vi "Login.vi"(5 "key":string="pGHs5Pd97hphPAMAKeEquwhT8aC4MC2e", 7 "userid":string="ADMIN", 8 "Error In":errorcluster, 9 "Command to webservice":string(combo)="https://iken.sasken.com/", 10 "password":string="123456Aa#", 11 "IN HTTPS client handle":T1) -> (0 "Error Out":errorcluster, 1 "Header of response":string, 2 "Body of reponse":string, 3 "OUT HTTPS client handle":T1, 4 "Response time":u32)   [LabVIEW 2017]
doc: "LOGIN SubVI\nThis SubVI is capable to login to webserver with user name and password and provides the reponse from webserver to user\nwith status code and sid. So user can utilise these two values status code and sid in his test case for validating the test case, is pass or fail.\n\nFinal testcase verdict pass or fail is validated with status code 0,1,2,3,4, so on...27 response recieved from webserver, Status code is validated with ini file located at global folder location, user can configure status code if any changes in future and it is located at\n\nC:\\Integration_Workspace\\Test_Component\\Ultrasonic_Test_Scripts\\Build\\UltraSonic_Test_Scripts\\Generic_Common\\Webserver\\StatusCodes.ini"
uses:
  <vilib>/httpClient/ClientHandle.ctl
  <vilib>/httpClient/POSTBuffer.vi
  <vilib>/httpClient/LabVIEWHTTPClient.lvlib
panel:
  # "RESPONSE FROM THE WEBSERVER"
  # "LOGIN TO WEBSERVER"
  # "ERROR"
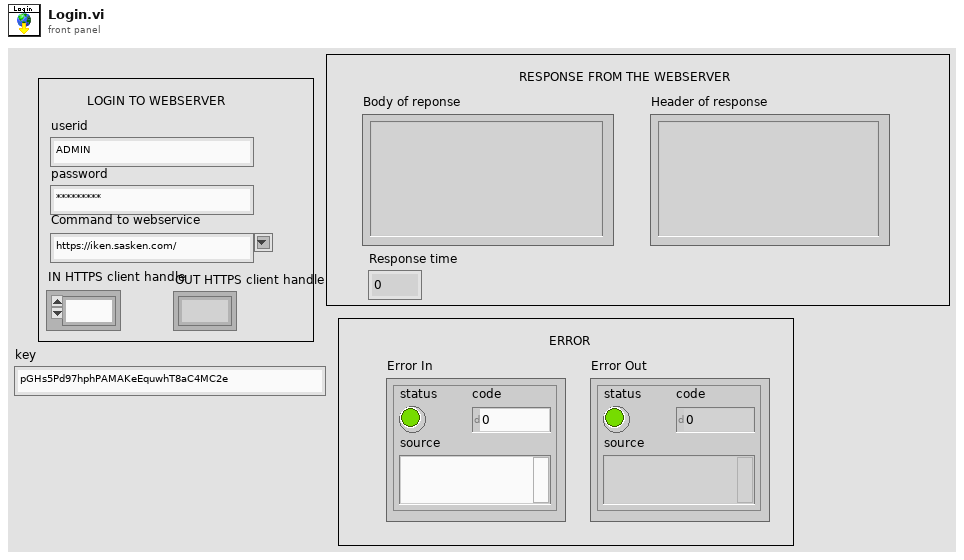
[diagram p1: front panel]
types:
  T1 = typedef "LabVIEWHTTPClient.lvlib/ClientHandle.ctl" = refnum<k1>
  T2 = cluster{"userid ":string, "password":string, "key":string}
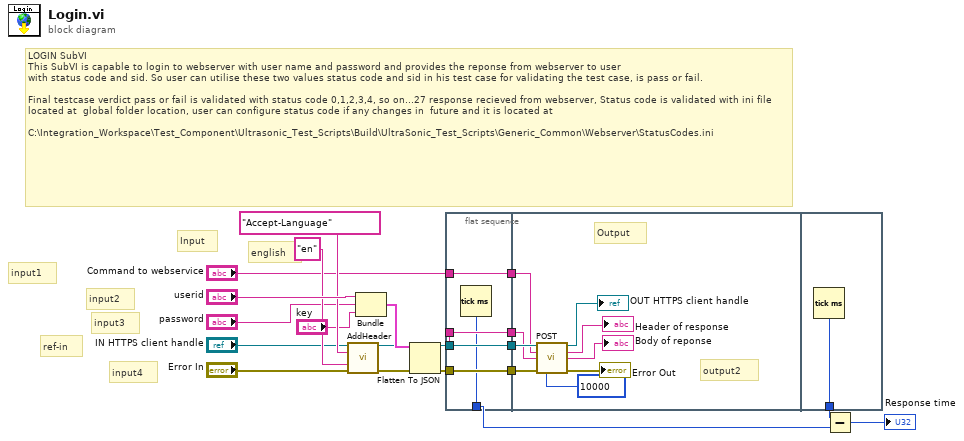
[diagram p0: block diagram]
diagram:
  # "input4"
  # "ref-in"
  # "input3"
  # "input2"
  # "input1"
  # "LOGIN SubVI\nThis SubVI is capable to login to webserver with user name and password and provides the reponse from webserver to user\nwith status code and sid. So user can utilise these two values status code and sid in his test case for validating the test case, is pass or fail.\n\nFinal testcase verdict pass or fail is validated with status code 0,1,2,3,4, so on...27 response recieved from webserver, Status code is validated with ini file located at  global folder location, user can configure status code if any changes in  future and it is located at\n\nC:\\Integration_Workspace\\Test_Component\\Ultrasonic_Test_Scripts\\Build\\UltraSonic_Test_Scripts\\Generic_Common\\Webserver\\StatusCodes.ini"
  # "Input"
  # "english"
  n1 = call <vilib>:"AddHeader.vi"("client handle"="IN HTTPS client handle", "header"="Accept-Language", "value"="en", "error in (no error)"="Error In") -> ("client handle out"=w12:T1, "error out"=w19:errorcluster)  [unwired: 10 in]
  n2 = Bundle("userid"="userid", "password"="password", "key"="key") -> (w16:T2)  [unwired: 1 in]
  n3 = Flatten To JSON(anything=w16, error in (no error)=w19) -> (JSON string=w9:string, 11:w11:errorcluster)  [unwired: 1 in]
  n4 = flat-sequence {
    tunnel: w9 -> [w22]
    tunnel: "Command to webservice" -> [w23]
    tunnel: w11 -> [w24]
    tunnel: w12 -> [w25]
    tunnel: [w25] -> w8
    tunnel: [w24] -> w7
    tunnel: [w23] -> w6
    tunnel: [w22] -> w5
    tunnel: [w21] -> w4
    tunnel: w8 -> [w32]
    tunnel: w7 -> [w31]
    tunnel: w6 -> [w30]
    tunnel: w5 -> [w29]
    tunnel: [w35] -> w3
    frame #0 {
      n5 = Tick Count (ms)() -> (millisecond timer value=w21:u32)
    }
    frame #1 {
      # "output2"
      # "Output"
      n6 = call-poly <vilib>:"POST.vi"("client handle"=w32, "url"=w30, "buffer"=w29, "error in (no error)"=w31, "timeout (10000)"=10000) -> ("client handle out"=→"OUT HTTPS client handle":T1, "headers"=→"Header of response":string, "body"=→"Body of reponse":string, "error out"=→"Error Out":errorcluster)  [unwired: 7 in]
    }
    frame #2 {
      n7 = Tick Count (ms)() -> (millisecond timer value=w35:u32)
    }
  }
  n8 = Subtract(x=w3, y=w4) -> (x-y=→"Response time":u32)
